vi "Robot Global Data.vi"() -> ()   [LabVIEW 2019]
doc: "This global VI can contain as many global variables as you need. Place a control on the panel, give it a good name. To read or write to it from a VI, drag the icon to the diagram of that VI. You can also drag from the project. Click on the node to change which global you access. You shouldn't have multiple locations writing to a global or it will cause a race-condition."
uses:
  <vilib>/Rock Robotics/WPI/Camera/WPI_CameraImageSize.ctl
  <vilib>/Rock Robotics/WPI/DriverStation/WPI_DriverStationRobotMode2.ctl
panel:
  out "PoseEstUpdateErr":bool
  out "PoseEstNewErr":bool
  out "PoseEst_PoseAng_RAD":dbl format="%22_5f"
  out "PoseEst_PoseY_M":dbl format="%22_5f"
  out "PoseEst_PoseX_M":dbl format="%22_5f"
  out "Ctrl_Loop_PoseEst_UpdateTime_Avg_MS":dbl format="%22_5f"
  out "Ctrl_Loop_PoseEst_AvgTime_MS":dbl format="%22_5f"
  out "Ctrl_Loop_PoseEst_Time_MS":dbl format="%22_5f"
  out "Gyro_DEG":dbl format="%22_5f"
  out "Ctrl_Loop_Main_OdomTime_Avg_MS":dbl format="%22_5f"
  out "Ctrl_Loop_Main_AvgTime_MS":dbl format="%22_5f"
  out "Ctrl_Loop_Main_Time_MS":dbl format="%22_5f"
  out "Odom_PoseAng_RAD":dbl format="%22_5f"
  out "Odom_PoseY_M":dbl format="%22_5f"
  out "Odom_PoseX_M":dbl format="%22_5f"
  in  "Robot Mode":T1
  in  "image size":T2=enum."320x240"
  in  "Enable Vision":bool
  # "Odometry..."
  # "PoseEst"
  # "Main Control Loop Time"
  # "State Space Pose Est Loop Time"
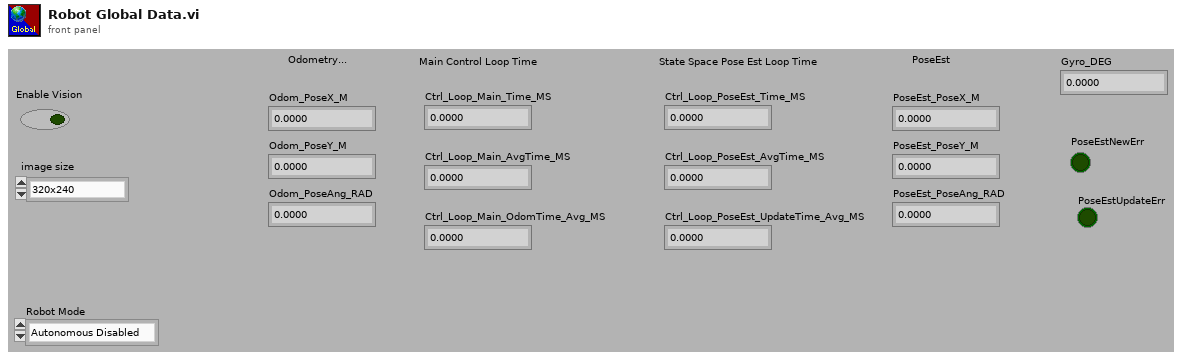
[diagram p1: front panel]
types:
  T1 = typedef "WPI_DriverStationRobotMode2.ctl" = enum16{"Autonomous Disabled", "Autonomous Enabled", "Teleop Disabled", "Teleop Enabled", "Disconnected", "Finish", "Test Disabled", "Test Enabled", "Emergency Stopped"}
  T2 = typedef "WPI_CameraImageSize.ctl" = enum16{"640x480", "320x240", "160x120", "Custom"}
diagram:
